vi "Emballage_BDD_lecture_CODE_GESTION.vi"(8 "Error in":errorcluster caption="Error in (no error)", 10 "NOVALVE_FILTRE":string, 11 "ID_ARTICLE_GPAO":string) -> (0 "Error out":errorcluster, 3 "données":string[](array[string]))   [LabVIEW 2020]
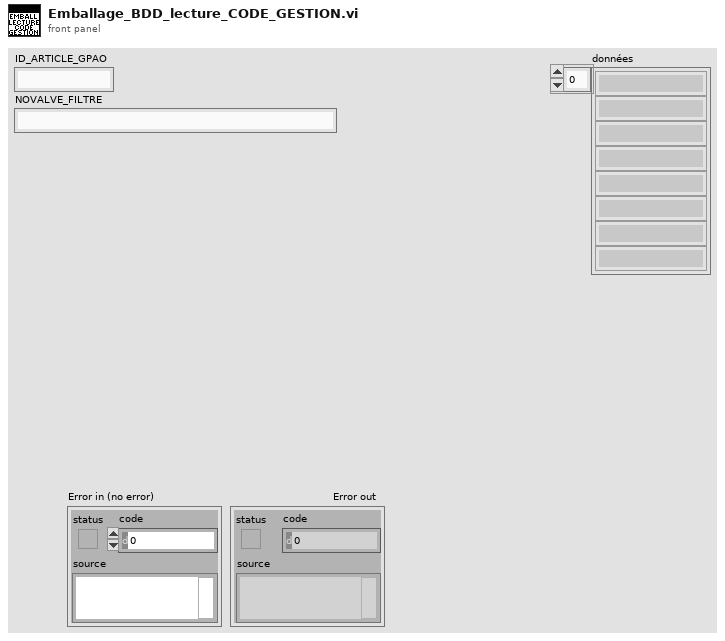
[diagram p1: front panel]
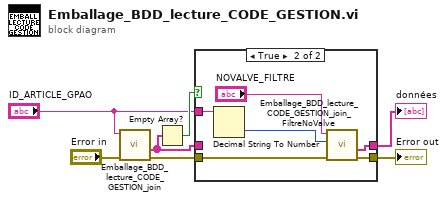
[diagram p0: block diagram]
diagram:
  n1 = call "Emballage_BDD_lecture_CODE_GESTION_join.vi"("error in"="Error in", "ID_ARTICLE_GPAO"="ID_ARTICLE_GPAO") -> ("error out"=w5:errorcluster, "données"=w2:string[])  [unwired: 6 in, 2 out]
  n2 = Empty Array?(array=w2) -> (empty?=w7:bool)
  n3 = case shown="True" w7 {
    tunnel: w5 -> [w9 w14]
    tunnel: [w9 w13] -> w4
    tunnel: [w8 w12] -> w3
    tunnel: w2 -> [w8 _]
    tunnel: "ID_ARTICLE_GPAO" -> [_ w11]
    frame False {
    }
    frame True {
      n4 = Decimal String To Number(string=w11) -> (number=w10:i32)  [unwired: 2 in, 1 out]
      n5 = call "Emballage_BDD_lecture_CODE_GESTION_join_FiltreNoValve.vi"("error in"=w14, "ID_ARTICLE"=w10, "NOVALVE_FILTRE"="NOVALVE_FILTRE") -> ("error out"=w13:errorcluster, "données Final"=w12:string[])  [unwired: 5 in, 2 out]
    }
  }
  "Error out" <- w4
  "données" <- w3
